vi "Get Device Identification.vi"(8 "error in (no error)":errorcluster, 11 "NRT8000 in":refnum<class "NRT8000.lvclass">) -> (0 "error out":errorcluster, 1 "Firmware Revision":string, 2 "Serial Number":string, 3 "NRT8000 out":refnum<class "NRT8000.lvclass">, 4 "Device Name":string, 5 "Manufacturer Name":string)   [LabVIEW 2018, in "NRT8000.lvlib" / "NRT8000.lvclass"]
uses:
  NRT8000.lvclass
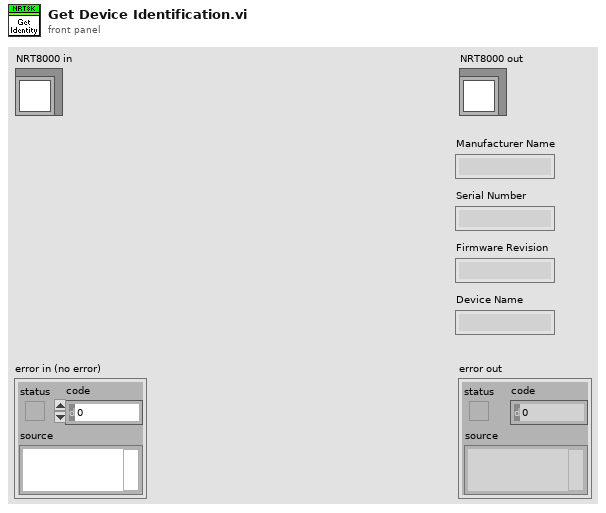
[diagram p1: front panel]
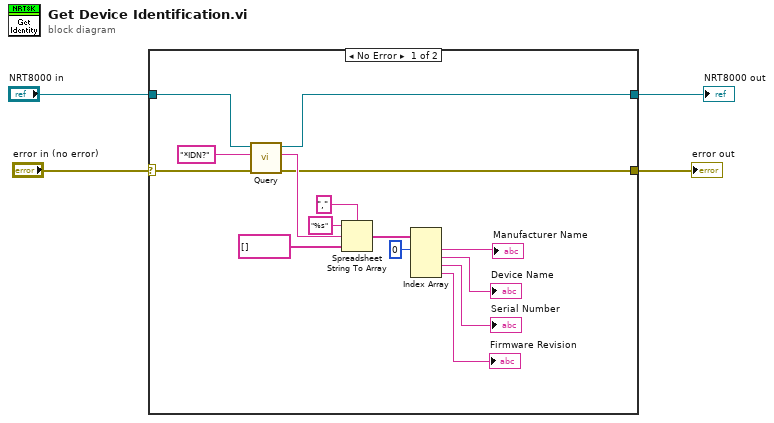
[diagram p0: block diagram]
diagram:
  n1 = case shown="No Error" "error in (no error)" {
    selector: "error in (no error)" -> [w19 w21]
    tunnel: [w5 w21] -> w3
    tunnel: [w16 w20] -> w2
    tunnel: "NRT8000 in" -> [w17 w20]
    frame No Error {
      n2 = call "Query.vi"("error in (no error)"=w19, "Cmd"="*IDN?", "NRT8000 in"=w17) -> ("error out"=w5:errorcluster, "Rsp"=w14:string, "NRT8000 out"=w16:refnum<class "NRT8000.lvclass">)  [unwired: 6 in]
      n3 = Spreadsheet String To Array(delimiter (Tab)=",", format string="%s", spreadsheet string=w14, array type (2D Dbl)=string[] []) -> (array=w11:string[])
      n4 = Index Array(array=w11, index #1=0 ("index")) -> (element #1=→"Manufacturer Name":string, element #2=→"Device Name":string, element #3=→"Serial Number":string, element #4=→"Firmware Revision":string)  [unwired: 3 in]
    }
    frame Error {
    }
  }
  "error out" <- w3
  "NRT8000 out" <- w2
